vi "startSnapping.vi"(8 "error in (no error)":errorcluster, 9 "releaseWhenReady":bool, 11 "CameraManager in":refnum<class "CameraManager.lvclass">) -> (0 "error out":errorcluster, 3 "CameraManager out":refnum<class "CameraManager.lvclass">)   [LabVIEW 2009, in "iManagement.lvlib" / "CameraManager.lvclass"]
uses:
  CameraManager.lvclass
  CameraManager.lvclass/CameraManager.ctl
  Hal/Channels/Camera/CameraController.lvclass
  Hal/Channels/Camera/CameraEventsManager/CameraEventsManger.lvclass
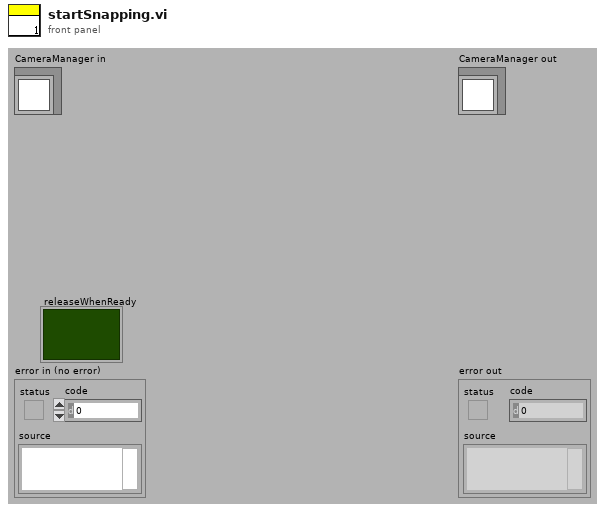
[diagram p1: front panel]
types:
  T1 = cluster{"frontEndEvents":cluster{"snapShotEvent":refnum<user-event>, "stopShooting":refnum<user-event>, "userSnapShot":refnum<user-event>}, "backEndEvents":cluster{"picture":refnum<user-event>}}
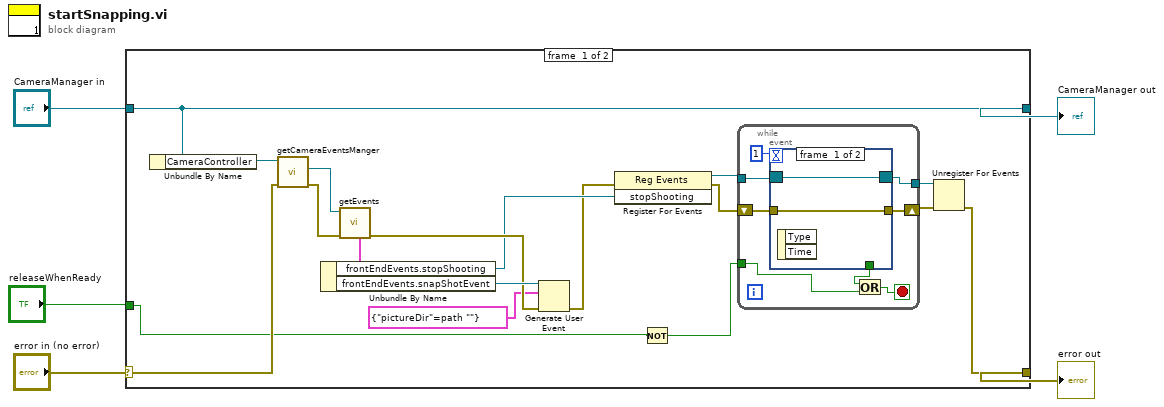
[diagram p0: block diagram]
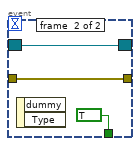
[diagram p2: hidden frame]
diagram:
  n1 = case shown="No Error" "error in (no error)" {
    selector: "error in (no error)" -> [w19 w38]
    tunnel: [w8 w38] -> w4
    tunnel: [w23 w37] -> w2
    tunnel: "CameraManager in" -> [w23 w37]
    tunnel: "releaseWhenReady" -> [w7 _]
    frame #0 {
      n2 = Unbundle By Name(w23) -> ("CameraController"=w20:refnum<class "CameraController.lvclass">)
      n3 = call-dynamic "getCameraEventsManger.vi"("error in (no error)"=w19, "CameraController.lvclass in"=w20) -> ("error out"=w21:errorcluster, "Hardware:Channels.lvlib:CameraEventsManger.lvclass"=w22:refnum<class "CameraEventsManger.lvclass">)  [unwired: 7 in, 1 out]
      n4 = call-dynamic "getEvents.vi"("error in (no error)"=w21, "CameraEventsManger in"=w22) -> ("error out"=w16:errorcluster, "snapperEvents"=w18:T1)  [unwired: 5 in, 3 out]
      n5 = Unbundle By Name(w18) -> ("frontEndEvents.stopShooting"=w14:refnum<user-event>, "frontEndEvents.snapShotEvent"=w17:refnum<user-event>)
      n6 = Generate User Event(user event=w17, event data cluster=cluster{"pictureDir":path} {"pictureDir"=path ""} ("event data"), error in=w16) -> (error out=w12:errorcluster)  [unwired: 1 out]
      n7 = register-events(error in=w12, w14) -> (reference out=w13:refnum<event-registration>, error out=w11:errorcluster)  [unwired: 1 in]
      n8 = Not(x=w7) -> (.not. x?=w6:bool)
      n9 = while {
        tunnel: w13 -> [w29]
        shift-right: [w30] -> w10
        shift-left: w11 -> [w31]
        tunnel: [w28] -> w9
        tunnel: w6 -> [w25]
        stop <- w24 stop-if-true
        n10 = event shown="[1] <stopShooting>: User Event" {
          selector: w29 -> [w32 w34]
          dyn-events: [w32 w34] -> w28
          timeout: 1 -> [_ _]
          tunnel: w31 -> [w33 w35]
          tunnel: [w33 w35] -> w30
          tunnel: [_ TRUE] -> w26
          event #0 {
            n11 = event-data() -> ()  [unwired: 1 in, 2 out]
          }
          event #1 {
            n12 = event-data() -> ()  [unwired: 1 in, 2 out]
          }
        }
        n13 = Or(x=w26, y=w25) -> (x .or. y?=w24:bool)
      }
      n14 = Unregister For Events(event registration refnum=w9, error in=w10) -> (error out=w8:errorcluster)
    }
    frame #1 {
    }
  }
  "error out" <- w4
  "CameraManager out" <- w2
